vi "Get Last Error.vi"(8 "error in":errorcluster) -> (0 "error out":errorcluster)   [LabVIEW 2018, in "PCANBasic.lvlib" / "Win32 Event.lvclass"]
uses:
  Win32 Event.lvclass
  PCANBasic.lvlib
panel:
  out "Last Error":u32
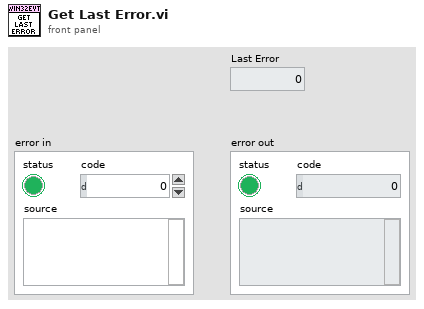
[diagram p1: front panel]
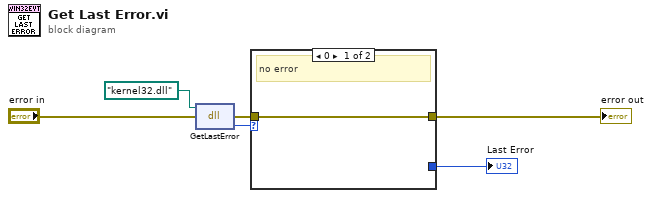
[diagram p0: block diagram]
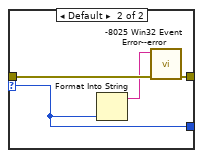
[diagram p2: hidden frame]
diagram:
  n1 = dll-call lib="?" fn="GetLastError"(path in=path "kernel32.dll", error in="error in") -> (error out=w1:errorcluster, "error"=w2:u32)  [unwired: 1 in, 1 out]
  n2 = case shown="0" w2 {
    selector: w2 -> [_ w8]
    tunnel: w1 -> [w7 w11]
    tunnel: [w7 w9] -> w5
    tunnel: [_ w8] -> w4
    frame 0 {
      # "no error"
    }
    frame Default {
      n3 = Format Into String(w8) -> (resulting string=w10:string)  [unwired: 3 in, 1 out]
      n4 = call "-8025 Win32 Event Error--error.vi"("error in"=w11, "Argument"=w10) -> ("error out"=w9:errorcluster)  [unwired: 8 in, 1 out]
    }
  }
  "error out" <- w5
  "Last Error" <- w4
